vi "Create All Message Queues.vi"(8 "error in (no error)":errorcluster) -> (0 "error out":errorcluster, 2 "User Events":T1, 3 "Queues out":T2)   [LabVIEW 2017, in "Message Queue.lvlib"]
doc: "This VI creates and initializes all the message queues for your application. If your application requires more than one message queue, right-click the \"Message Queues\" constant above and select Open Type Def. Add the new Message Queue(s) to the type definition, then initialize them in this VI."
uses:
  Message Queue.lvlib
  All Message Queues.ctl
  Message Cluster.ctl
  Configuration/Controls/Config Commands.ctl
  Configuration/Controls/ConfigStates.ctl
  Elevator/Controls/Elevator Command Event.ctl
  Elevator/Controls/Elevator Commands.ctl
  Controls/User Events.ctl
  Error Handler/Controls/Error EventData.ctl
  Error Handler/Controls/Error Type.ctl
  User Events/User Events.lvlib
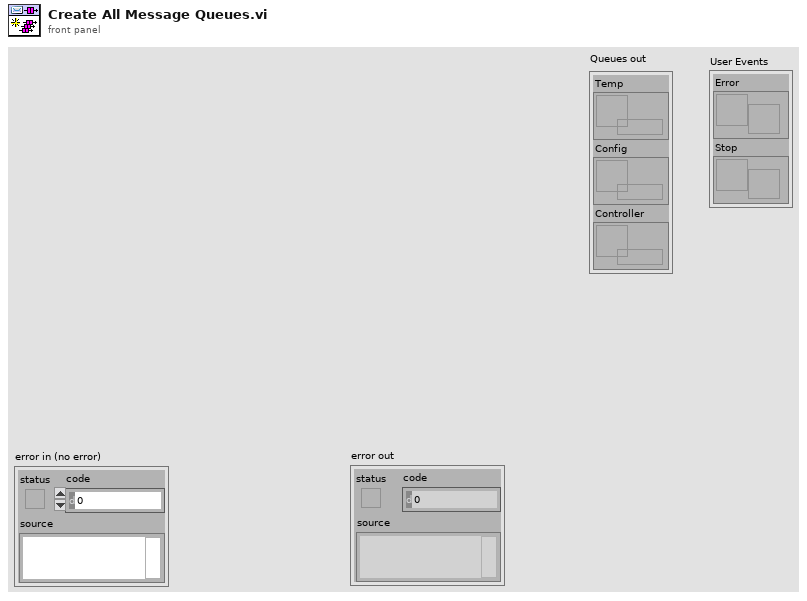
[diagram p1: front panel]
types:
  T1 = typedef "User Events.ctl" = cluster{"Error":refnum<user-event>, "Stop":refnum<user-event>}
  T2 = typedef "Message Queue.lvlib/All Message Queues.ctl" = cluster{"Temp":refnum<queue>, "Config":refnum<queue>, "Controller":refnum<queue>}
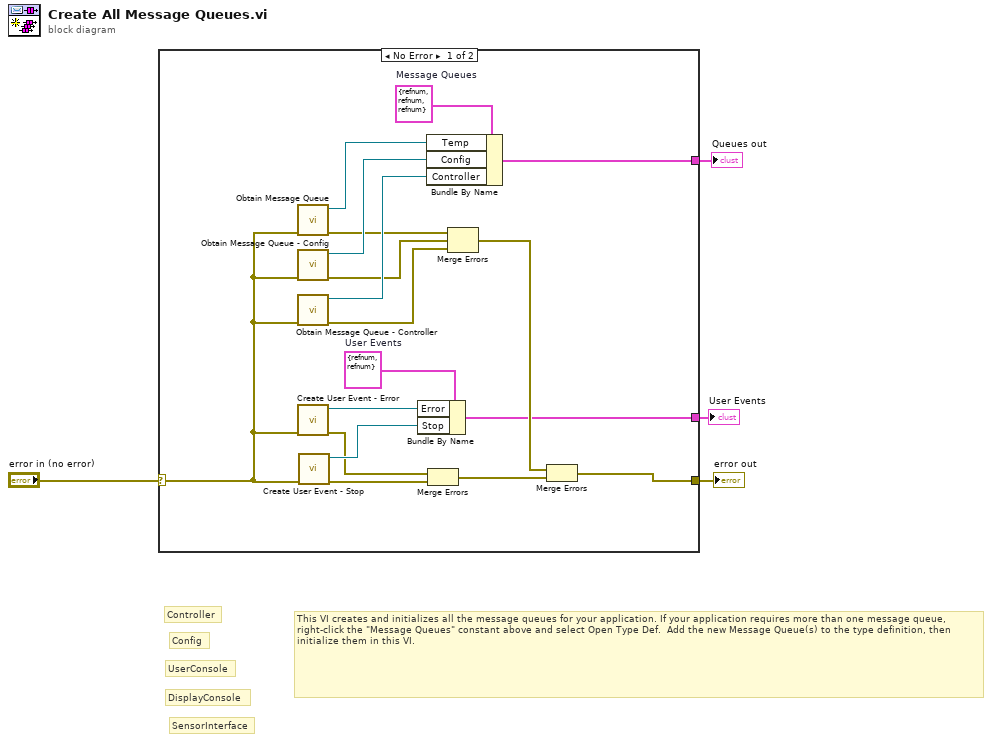
[diagram p0: block diagram]
diagram:
  # "SensorInterface"
  # "DisplayConsole"
  # "UserConsole"
  # "Config"
  # "Controller"
  # "This VI creates and initializes all the message queues for your application. If your application requires more than one message queue, right-click the \"Message Queues\" constant above and select Open Type Def.  Add the new Message Queue(s) to the type definition, then initialize them in this VI."
  n1 = case shown="No Error" "error in (no error)" {
    selector: "error in (no error)" -> [w14 w23]
    tunnel: [w6 w23] -> w4
    tunnel: [w21 _] -> w3
    tunnel: [w5 _] -> w1
    frame No Error {
      w13 = T1 {"Error"=refnum, "Stop"=refnum}  # User Events
      w22 = T2 {"Temp"=refnum, "Config"=refnum, "Controller"=refnum}  # Message Queues
      n2 = call "Obtain Message Queue.vi"("error in (no error)"=w14) -> ("error out"=w17:errorcluster, "Message Queue"=w20:refnum<queue>)  [unwired: 9 in]
      n3 = call "Obtain Message Queue - Config.vi"("error in (no error)"=w14) -> ("error out"=w16:errorcluster, "Config"=w19:refnum<queue>)  [unwired: 9 in]
      n4 = call "Obtain Message Queue - Controller.vi"("error in (no error)"=w14) -> ("error out"=w15:errorcluster, "Controller"=w18:refnum<queue>)  [unwired: 9 in]
      n5 = call "Create User Event - Error.vi"("error in (no error)"=w14) -> ("error out"=w9:errorcluster, "UE Error"=w12:refnum<user-event>)  [unwired: 9 in]
      n6 = call "Create User Event - Stop.vi"("error in (no error)"=w14) -> ("error out"=w10:errorcluster, "User Event - Stop"=w11:refnum<user-event>)  [unwired: 9 in]
      n7 = Bundle By Name(cluster=w13, "Error"=w12, "Stop"=w11) -> (w5:T1)
      n8 = Bundle By Name(cluster=w22, "Temp"=w20, "Config"=w19, "Controller"=w18) -> (w21:T2)
      n9 = Merge Errors(w9, w10) -> (w8:errorcluster)
      n10 = Merge Errors(w17, w16, w15) -> (w7:errorcluster)
      n11 = Merge Errors(w7, w8) -> (w6:errorcluster)
    }
    frame Error {
    }
  }
  "Queues out" <- w3
  "error out" <- w4
  "User Events" <- w1
